vi "Method.vi"(4 "Value":refnum<class "Abs_Complex Double Float.lvclass">) -> (1 "Result":refnum<class "Abs_Boolean.lvclass">)   [LabVIEW 2021, in "Not Equal 0_CPLX_DBL.lvclass"]
uses:
  Not Equal 0_CPLX_DBL.lvclass
  Abs_Types/Complex Double Float/Abs_Complex Double Float.lvclass
  Abs_Types/Boolean/Abs_Boolean.lvclass
  C:/TSA/LV_Abstract/Source/Functions/Support/Compare/One Term/CPLX_DBL/AbsComp_One Term_CPLX_DBL.lvclass
  C:/Program Files (x86)/National Instruments/LabVIEW 2021/vi.lib/TSA/Abstract Data Classes/Abs_Types/Boolean/Abs_Boolean.lvclass
  Support/Compare/One Term/CPLX_DBL/AbsComp_One Term_CPLX_DBL.lvclass/AbsComp_One Term_CPLX_DBL.ctl
  Support/Compare/One Term/CPLX_DBL/Properties/Write Numeric A.vi
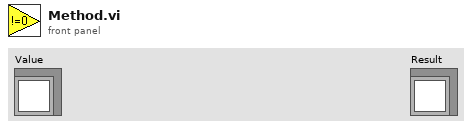
[diagram p1: front panel]
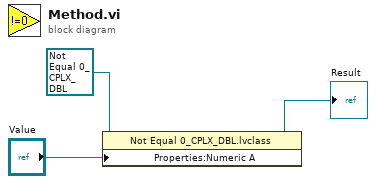
[diagram p0: block diagram]
diagram:
  n1 = property class="Not Equal 0_CPLX_DBL.lvclass"(reference=refnum<class "Not Equal 0_CPLX_DBL.lvclass"> refnum ("Greater 0_U64.lvclass"), "Properties:Numeric A"="Value") -> (reference out=→"Result":refnum<class "Not Equal 0_CPLX_DBL.lvclass">)  [unwired: 1 in, 1 out]
